vi "take_screenshot.vi"(4 "Visible area only? (f)":bool, 5 "error in (no error)":errorcluster, 6 "IMG_FORMAT":enum32{".png", ".jpg", ".bmp"}(ring), 7 "Image path":path, 8 "vi path":string) -> (0 "error out":errorcluster, 2 "Image path":path)   [LabVIEW 2018]
doc: "This example captures an image of the front panel of a VI and saves the image to a JPG, PNG, or BMP file."
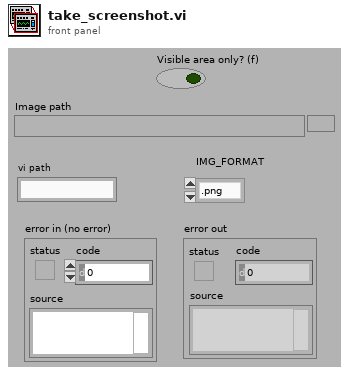
[diagram p1: front panel]
types:
  T1 = typedef "imagedata.ctl" = cluster{"image type":i32, "image depth":i32, "image":u8[], "mask":u8[], "colors":u32[], "Rectangle":cluster{"left":i16, "top":i16, "right":i16, "bottom":i16}}
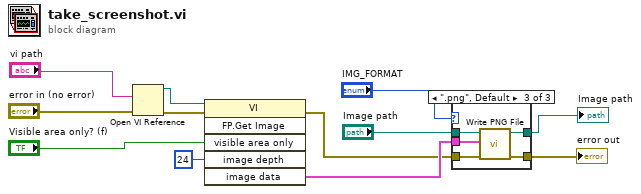
[diagram p0: block diagram]
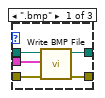
[diagram p2: hidden frame]
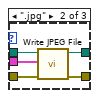
[diagram p3: hidden frame]
diagram:
  n1 = Open VI Reference(vi path="vi path", error in (no error)="error in (no error)") -> (vi reference=w12:refnum<vi>, error out=w10:errorcluster)  [unwired: 4 in]
  n2 = invoke class="VI" method="FP.Get Image"(reference=w12, error in=w10, "visible area only"="Visible area only? (f)", "image depth"=24 ("Image Depth")) -> (error out=w9:errorcluster, "image data"=w11:T1)  [unwired: 2 in, 4 out]
  n3 = case shown="\".png\", Default" "IMG_FORMAT" {
    tunnel: w11 -> [w16 w21 w26]
    tunnel: w9 -> [w15 w22 w27]
    tunnel: "Image path" -> [w17 w20 w25]
    tunnel: [w14 w19 w24] -> w5
    tunnel: [w13 w18 w23] -> w4
    frame ".bmp" {
      n4 = call <vilib>:"Write BMP File.vi"("error in (no error)"=w15, "image data"=w16, "path to BMP file"=w17) -> ("error out"=w14:errorcluster, "path"=w13:path)  [unwired: 7 in]
    }
    frame ".jpg" {
      n5 = call <vilib>:"Write JPEG File.vi"("error in (no error)"=w22, "image data"=w21, "path to JPEG file"=w20) -> ("error out"=w19:errorcluster, "path"=w18:path)  [unwired: 7 in]
    }
    frame ".png", Default {
      n6 = call <vilib>:"Write PNG File.vi"("error in (no error)"=w27, "image data"=w26, "path to PNG file"=w25) -> ("error out"=w24:errorcluster, "path"=w23:path)  [unwired: 7 in]
    }
  }
  "error out" <- w5
  "Image path" <- w4
